vi "Add.vi"(8 "error in (no error)":errorcluster, 9 "Value":refnum<class>, 10 "Key":string, 11 "VariantAttribute in":refnum<class "MapImp.lvclass">) -> (0 "error out":errorcluster, 3 "VariantAttribute out":refnum<class "MapImp.lvclass">)   [LabVIEW 2013, in "LapDog.Collections.v_.Maps.lvlib" / "MapImp.lvclass"]
doc: "Add a key-value pair to the map.\n\nIf the key already exists, error 510202 is returned."
uses:
  MapImp.lvclass
  MapImp.lvclass/MapImp.ctl
  LapDog.Collections.Common/LapDog.Collections.v_.Common.lvlib
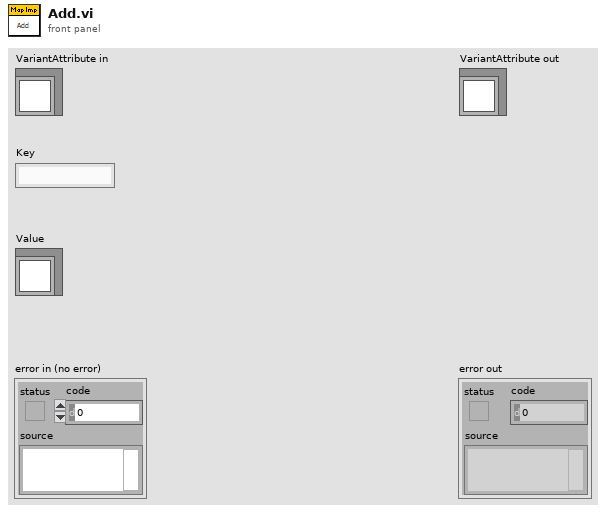
[diagram p1: front panel]
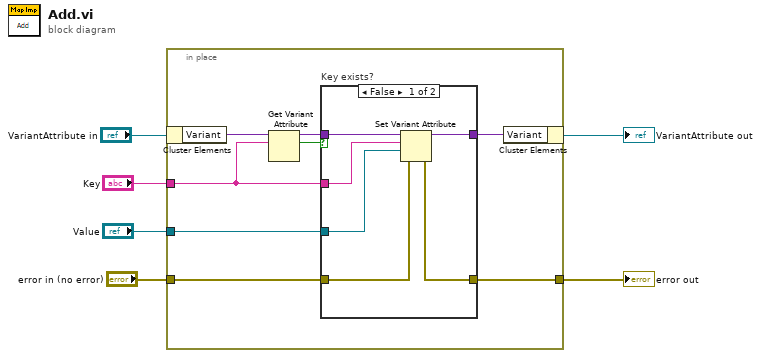
[diagram p0: block diagram]
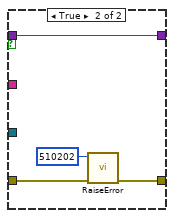
[diagram p2: hidden frame]
diagram:
  n1 = in-place {
    in-place-border: "Key" -> [w8]
    in-place-border: "error in (no error)" -> [w11]
    in-place-border: [w10] -> w3
    in-place-border: "Value" -> [w7]
    n2 = in-place-cluster #1("VariantAttribute in") -> ("Variant"=w14:variant)
    n3 = Get Variant Attribute(Variant=w14, name=w8) -> (duplicate Variant=w12:variant, found=w13:bool)  [unwired: 2 in, 2 out]
    n4 = case "Key exists?" shown="False" w13 {
      tunnel: w12 -> [w20 w21]
      tunnel: w11 -> [w18 w24]
      tunnel: [w17 w22] -> w10
      tunnel: [w19 w21] -> w9
      tunnel: w8 -> [w16 _]
      tunnel: w7 -> [w15 _]
      frame False {
        n5 = Set Variant Attribute(Variant=w20, name=w16, value=w15, error in=w18) -> (Variant out=w19:variant, error out=w17:errorcluster)  [unwired: 1 out]
      }
      frame True {
        n6 = call "RaiseError.vi"("error in (no error)"=w24, "Error Code"=510202) -> ("error out"=w22:errorcluster)  [unwired: 9 in]
      }
    }
    n7 = in-place-cluster #1("Variant"=w9) -> (→"VariantAttribute out":refnum<class "MapImp.lvclass">)
  }
  "error out" <- w3
